vi "N_Point_Running_Average.vi"(1 "n":i32, 2 "Input":dbl) -> (0 "Output":dbl)   [LabVIEW 2015]
uses:
  <vilib>/Analysis/baseanly.llb/Mean (DBL).vi
  <vilib>/Analysis/NI_AALBase.lvlib
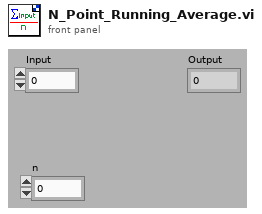
[diagram p1: front panel]
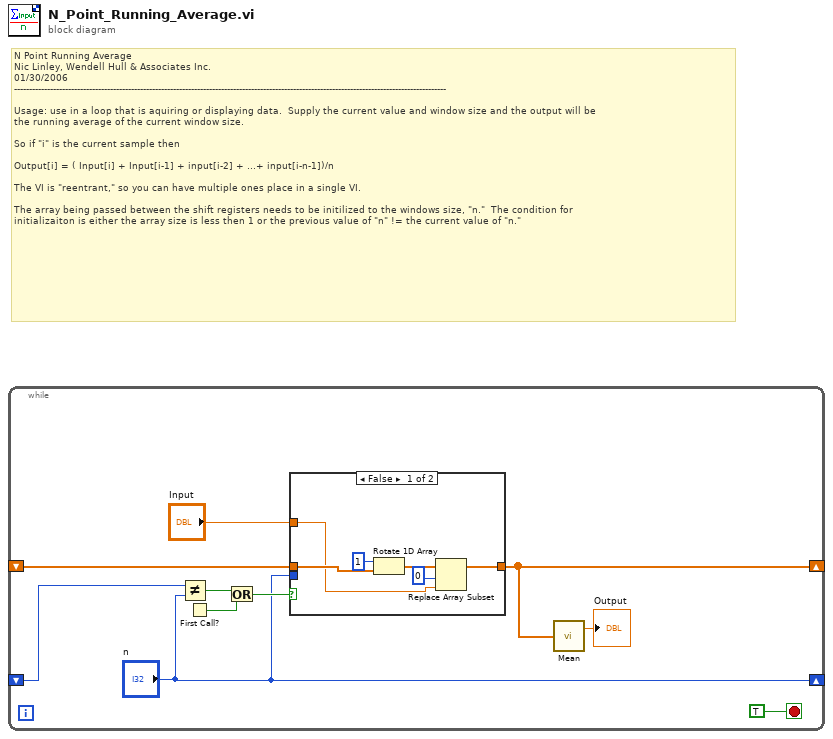
[diagram p0: block diagram]
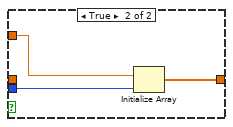
[diagram p2: hidden frame]
diagram:
  # "N Point Running Average \nNic Linley, Wendell Hull & Associates Inc.\n01/30/2006\n------------------------------------------------------------------------------------------------------------------------------------------------\n\nUsage: use in a loop that is aquiring or displaying data.  Supply the current value and window size and the output will be\nthe running average of the current window size.\n\nSo if \"i\" is the current sample then\n\nOutput[i] = ( Input[i] + Input[i-1] + input[i-2] + ...+ input[i-n-1])/n\n\nThe VI is \"reentrant,\" so you can have multiple ones place in a single VI.\n\nThe array being passed between the shift registers needs to be initilized to the windows size, \"n.\"  The condition for\ninitializaiton is either the array size is less then 1 or the previous value of \"n\" != the current value of \"n.\""
  n1 = while {
    shift-right: [w8] -> _
    shift-left: _ -> [w9]
    shift-right: ["n"] -> _
    shift-left: _ -> [w3]
    stop <- TRUE stop-if-true
    n2 = Not Equal?(x=w3, y="n") -> (x != y?=w2:bool)
    n3 = First Call?() -> (First Call?: T/F=w1:bool)
    n4 = Or(x=w2, y=w1) -> (x .or. y?=w5:bool)
    n5 = case shown="False" w5 {
      tunnel: "n" -> [_ w19]
      tunnel: "Input" -> [w11 w18]
      tunnel: [w16 w17] -> w8
      tunnel: w9 -> [w15 _]
      frame False {
        n6 = Rotate 1D Array(1:w15, 2:1 ("n")) -> (0:w14:dbl[])
        n7 = Replace Array Subset(array=w14, new element=w11, index=0) -> (w16:dbl[])
      }
      frame True {
        n8 = Initialize Array "Initialize Array"(w18, w19) -> (w17:dbl[])
      }
    }
    n9 = call-poly <vilib>:"Mean.vi"("X"=w8) -> ("mean"=→"Output":dbl)  [unwired: 1 out]
  }
